vi "Robot FPGA Utility Assign.vi"() -> ()   [LabVIEW 2014]
doc: "This FPGA VI defines the functionality that is needed for the C terminal connector for the myRIO sheepdog robot project. It provides two PWM outputs, two single-line counters (for the Hall effect encoders), and digital IO needed to command the motors. It also determines a measure of the derivative of the encoder counter lines (proportional to wheel speed)."
uses:
  <vilib>/Platform/TimedLoop/XDataNode/timing_clust.ctl
  <vilib>/Platform/TimedLoop/XDataNode/nitl_modes.ctl
  <vilib>/Platform/TimedLoop/XDataNode/wakeup.ctl
  <vilib>/rvi/Emulation/niFpgaSctlEmulationGetInTimedLoop.vi
  <vilib>/rvi/Emulation/niFpgaEmulationReportErrorSimple.vi
  <vilib>/rvi/Emulation/niFpgaGetClockAttributes.vi
  <vilib>/rvi/Emulation/niFpgaCriticalErrorInLSC.vi
  <vilib>/rvi/eio/common/nirviEmuTemplateMethod_errors.vi
  <vilib>/Platform/TimedLoop/XDataNode/XDataNode.xnode
  <vilib>/eio/EIONode/EIONode.xnode
  <vilib>/eio/EIOMethodNode/EIOMethodNode.xnode
  <vilib>/Platform/TimedLoop/XDataNode/XDNodeRunTimeDep.lvlib
panel:
  in  "Motor Dir 1":bool
  out "Encoder 1 Period":u32
  out "Encoder 1 Position":i16
  in  "Reset Encoder 1":bool
  in  "Duty Cycle Divisor":i16=30000
  in  "Duty Cycle 1":i16
  out "SYS.RDY":bool=TRUE
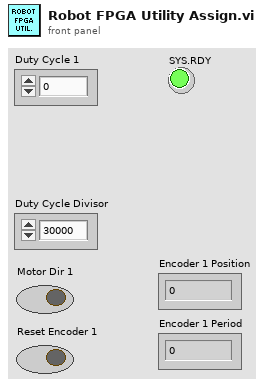
[diagram p1: front panel]
types:
  T1 = typedef "XDNodeRunTimeDep.lvlib/timing_clust.ctl" = cluster{"Expected End [f-1]":u64, "Actual End [f-1]":u64, "Finished Late? [f-1]":bool, "Expected End [i-1]":u64, "Actual End [i-1]":u64, "Finished Late? [i-1]":bool, "Expected Start [i]":u64, "Actual Start [i]":u64, "Expected Start [f]":u64, "Actual Start [f]":u64, "Source Name":string, "Structure Name":string, "Period":i64, "Deadline":i64, "Offset":i64, "Start":i64, "Priority":i32, "Timeout":i32, "Mode":T2, "Wakeup Reason":T3, "Error":errorcluster, "Source Type":string, "Secondary Source Type":string, "Global End Time":u64, "Global Start Time":u64, "Frame Duration":u64, "Iteration Duration":u64, "Assigned CPU":i32, "I/O Scan Engine Mode":u32}
  T2 = typedef "XDNodeRunTimeDep.lvlib/nitl_modes.ctl" = enum32{"No Change", "Process missed periods, maintain original phase", "Discard missed periods, maintain original phase", "Process missed periods, ignore original phase", "Discard missed periods, ignore original phase"}
  T3 = typedef "XDNodeRunTimeDep.lvlib/wakeup.ctl" = enum32{"Normal", "Aborted", "Asynchronous wakeup", "Timing source error", "Timed loop error", "Timeout"}
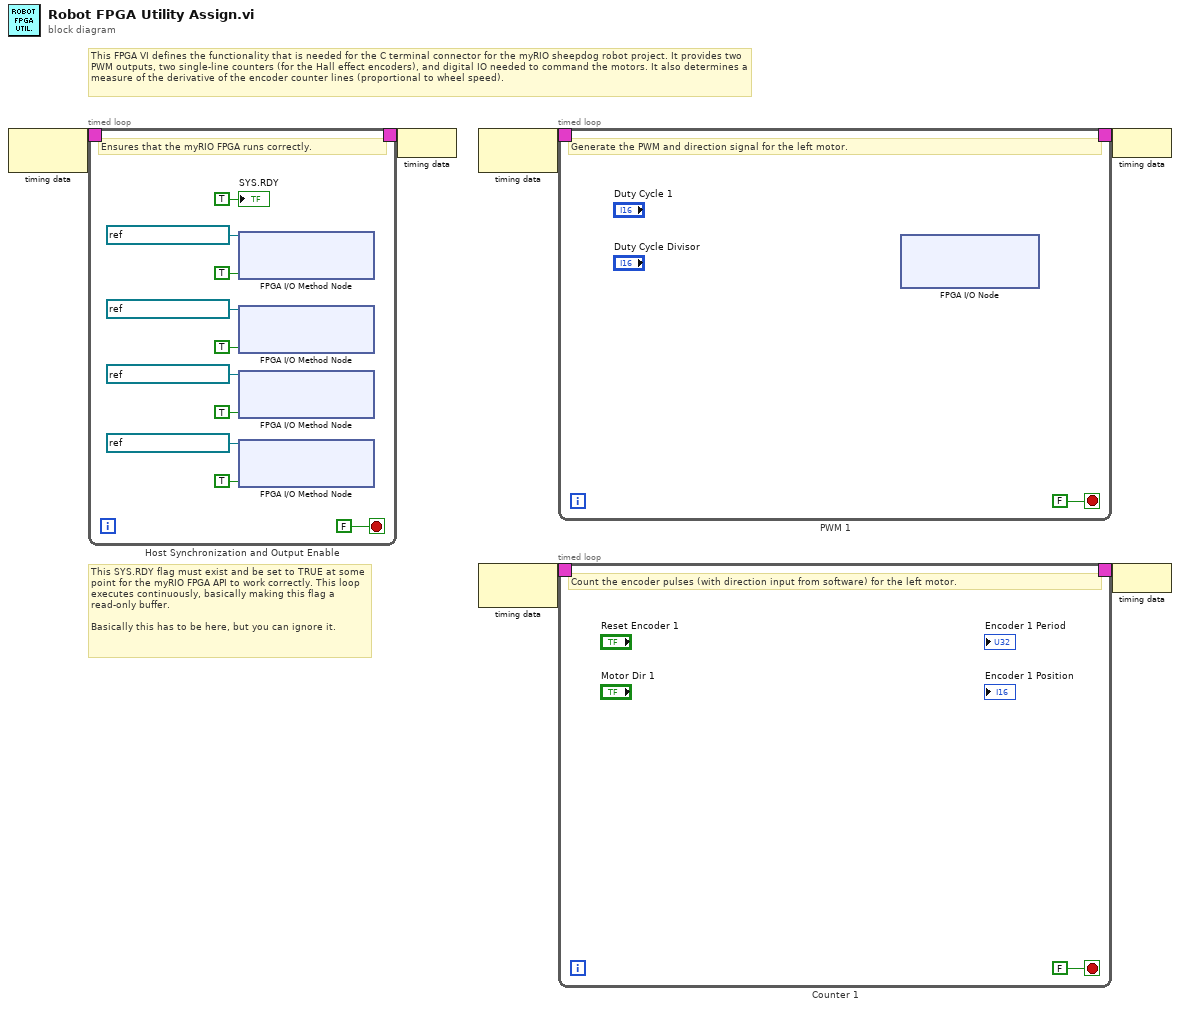
[diagram p0: block diagram]
diagram:
  # "This SYS.RDY flag must exist and be set to TRUE at some point for the myRIO FPGA API to work correctly. This loop executes continuously, basically making this flag a read-only buffer.\n\nBasically this has to be here, but you can ignore it."
  # "This FPGA VI defines the functionality that is needed for the C terminal connector for the myRIO sheepdog robot project. It provides two PWM outputs, two single-line counters (for the Hall effect encoders), and digital IO needed to command the motors. It also determines a measure of the derivative of the encoder counter lines (proportional to wheel speed)."
  n1 = node-c288() -> (w2:T1)  [unwired: 1 in]
  n2 = timed-loop "Host Synchronization and Output Enable" {
    timing: w2 -> [_]
    timing-out: [_] -> w1
    stop <- FALSE stop-if-true
    # "Ensures that the myRIO FPGA runs correctly."
    n3 = xnode "FPGA I/O Method Node"("FPGA I/O In"=refnum<k21> "ConnectorC/DIO1", "Enable"=TRUE) -> ()  [unwired: 1 out]
    n4 = xnode "FPGA I/O Method Node"("FPGA I/O In"=refnum<k21> "ConnectorC/DIO3", "Enable"=TRUE) -> ()  [unwired: 1 out]
    n5 = xnode "FPGA I/O Method Node"("FPGA I/O In"=refnum<k21> "ConnectorC/DIO5", "Enable"=TRUE) -> ()  [unwired: 1 out]
    n6 = xnode "FPGA I/O Method Node"("FPGA I/O In"=refnum<k21> "ConnectorC/DIO7", "Enable"=TRUE) -> ()  [unwired: 1 out]
    "SYS.RDY" <- TRUE
  }
  n7 = node-c288(w1) -> ()
  n8 = node-c288() -> (w6:T1)  [unwired: 1 in]
  n9 = node-c288() -> (w4:T1)  [unwired: 1 in]
  n10 = timed-loop "PWM 1" {
    timing: w6 -> [_]
    timing-out: [_] -> w5
    stop <- FALSE stop-if-true
    # "Generate the PWM and direction signal for the left motor."
    n11 = xnode "FPGA I/O Node"() -> ()  [unwired: 2 in, 4 out]
  }
  n12 = timed-loop "Counter 1" {
    timing: w4 -> [_]
    timing-out: [_] -> w3
    stop <- FALSE stop-if-true
    # "Count the encoder pulses (with direction input from software) for the left motor."
  }
  n13 = node-c288(w5) -> ()
  n14 = node-c288(w3) -> ()
